vi "Init.vi"(8 "error in (no error)":errorcluster, 11 "optimizer path":path=path "C:/Users/zachc/Documents/Reaction Rover/Plugins/Optimizers/Deep Reaction Optimizer/Source - zmq/start_inference.bat") -> (0 "error out":errorcluster, 3 "optimizer path (out)":path)   [LabVIEW 2020, in "Deep Reaction Optimizer Control Panel.lvlib"]
uses:
  Deep Reaction Optimizer Control Panel.lvlib
  Typedefs/Init.vi States.ctl
panel:
  in  "Connect Btn":bool
  # "1. Optimizer Start Script Path"
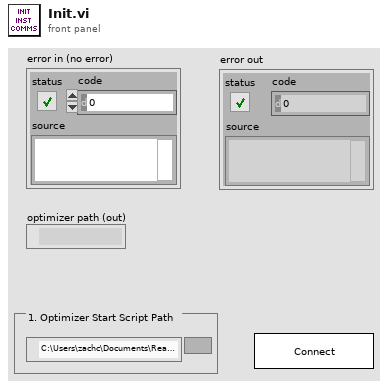
[diagram p1: front panel]
types:
  T1 = typedef "Deep Reaction Optimizer Control Panel.lvlib/Init.vi States.ctl" = enum16{"Waiting for connection", "Connecting", "Successful connection", "Failed to connect", "Closing"}
  T2 = enum32{"Invalid", "Standard", "Closed", "Hidden", "Minimized", "Maximized"}
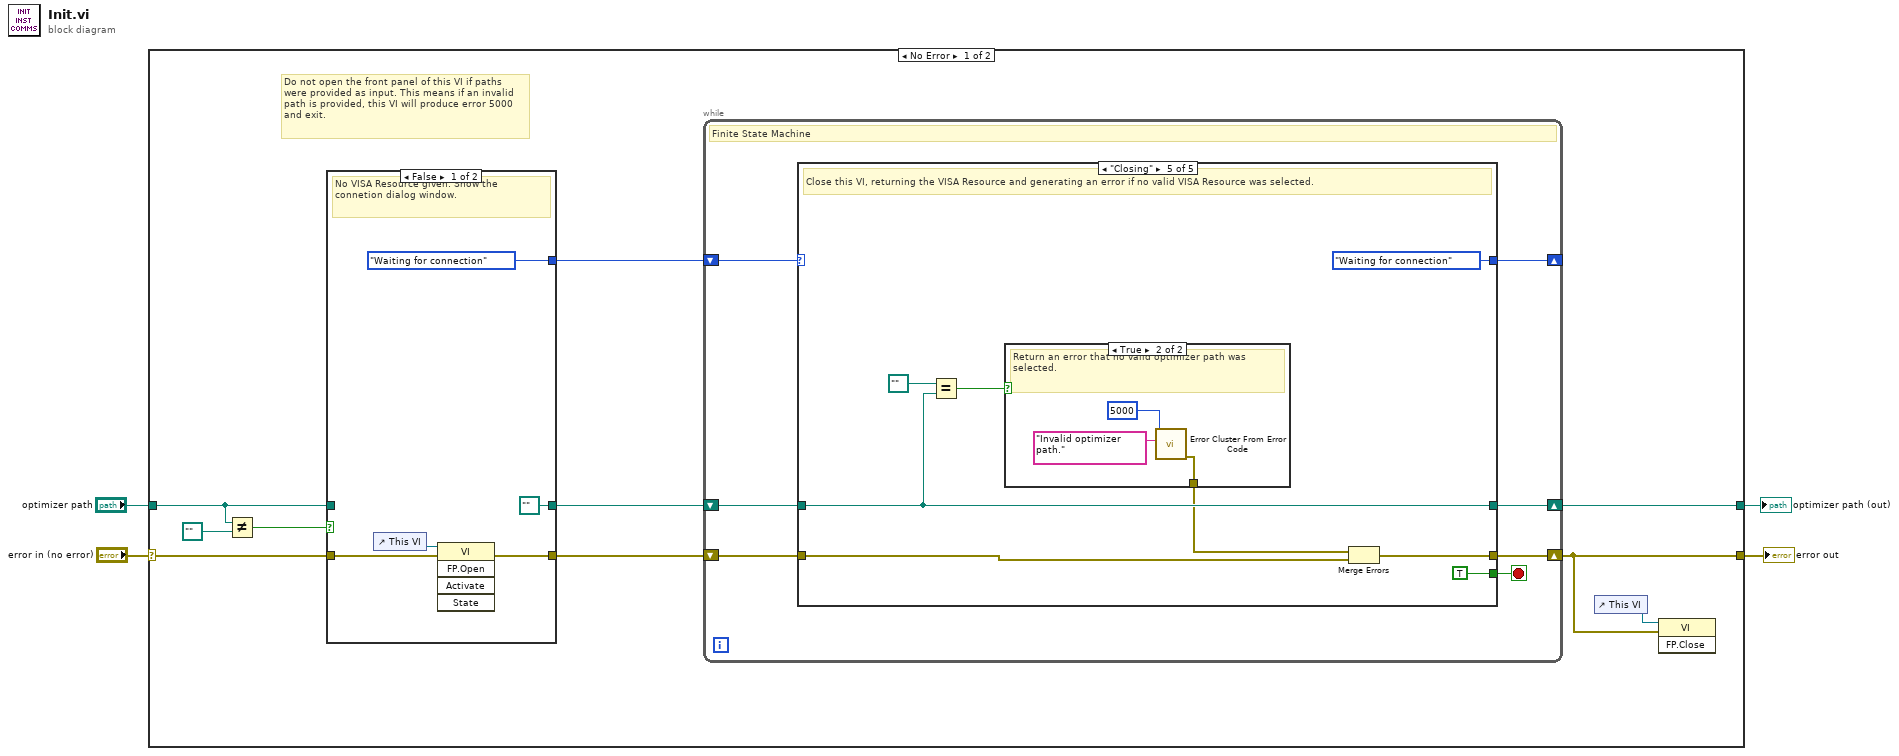
[diagram p0: block diagram]
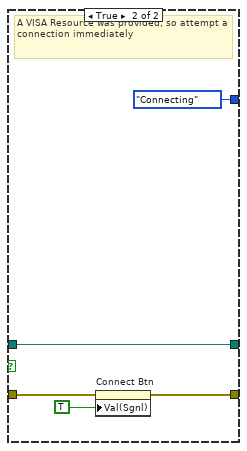
[diagram p2: hidden frame]
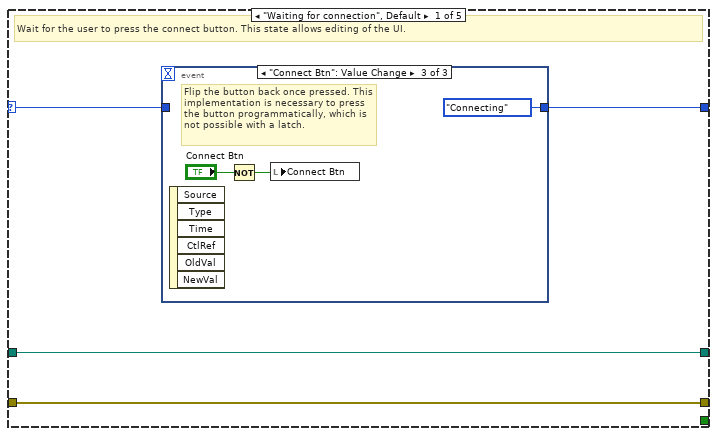
[diagram p3: hidden frame]
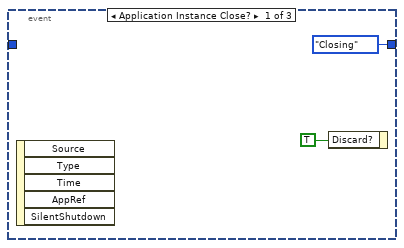
[diagram p4: hidden frame]
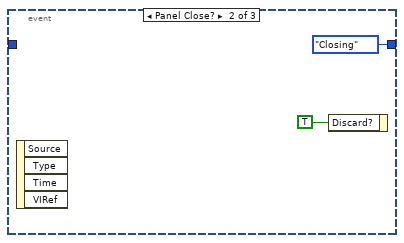
[diagram p5: hidden frame]
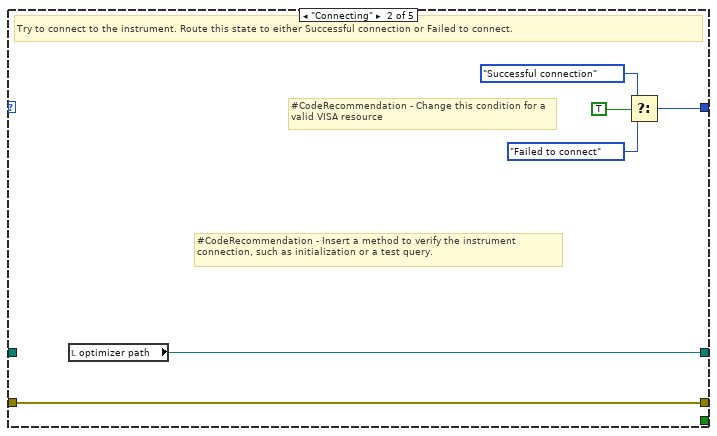
[diagram p6: hidden frame]
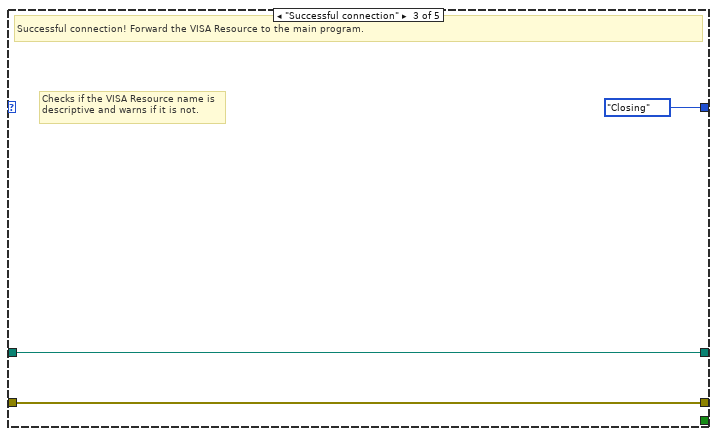
[diagram p7: hidden frame]
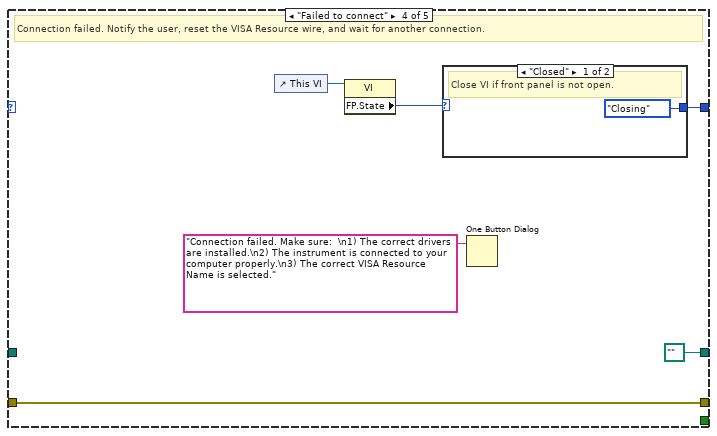
[diagram p8: hidden frame]
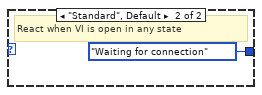
[diagram p9: hidden frame]
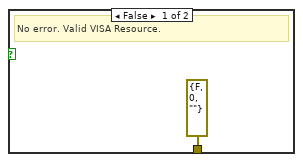
[diagram p10: hidden frame]
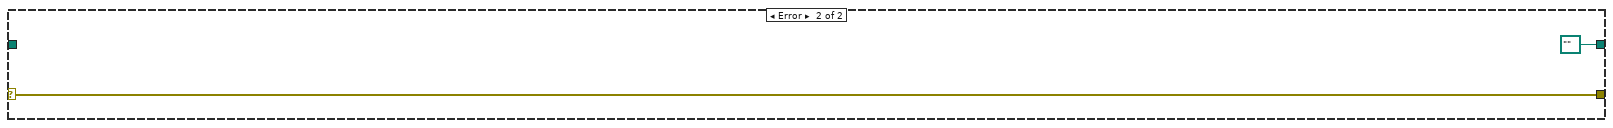
[diagram p11: hidden frame]
diagram:
  n1 = case shown="No Error" "error in (no error)" {
    selector: "error in (no error)" -> [w10 w73]
    tunnel: [w14 path "" ("VISA resource in")] -> w4
    tunnel: [w12 w73] -> w2
    tunnel: "optimizer path" -> [w6 _]
    frame No Error {
      # "Do not open the front panel of this VI if paths were provided as input. This means if an invalid path is provided, this VI will produce error 5000 and exit."
      n2 = Not Equal?(x=w6, y=path "" ("x")) -> (x != y?=w8:bool)
      n3 = case shown="False" w8 {
        tunnel: w10 -> [w18 w23]
        tunnel: [w17 w22] -> w9
        tunnel: [Init.vi_States."Waiting for connection" Init.vi_States."Connecting"] -> w7
        tunnel: w6 -> [_ w20]
        tunnel: [path "" ("optimizer path") w20] -> w5
        frame False {
          # "No VISA Resource given. Show the connetion dialog window."
          n4 = control-ref of="This VI"() -> (w19:refnum<vi>)
          n5 = invoke class="VI" method="FP.Open"(reference=w19, error in=w18) -> (error out=w17:errorcluster)  [unwired: 3 in, 4 out]
        }
        frame True {
          # "A VISA Resource was provided, so attempt a connection immediately"
          n6 = property on="Connect Btn" class="Bool (strict)"(error in=w23, "Val(Sgnl)"=TRUE) -> (error out=w22:errorcluster)  [unwired: 1 in, 1 out]
        }
      }
      n7 = while {
        shift-right: [w30] -> _
        shift-left: w7 -> [w31]
        shift-right: [w28] -> w14
        shift-left: w5 -> [w27]
        shift-right: [w25] -> w12
        shift-left: w9 -> [w26]
        stop <- w29 stop-if-true
        # "Finite State Machine"
        n8 = case shown="\"Closing\"" w31 {
          selector: w31 -> [w35 _ _ _ _]
          tunnel: [w34 w48 Init.vi_States."Closing" w57 Init.vi_States."Waiting for connection"] -> w30
          tunnel: [_ _ _ _ TRUE] -> w29
          tunnel: [w32 w43 w49 path "" ("VISA resource in") w64] -> w28
          tunnel: w27 -> [w32 _ w49 _ w64]
          tunnel: w26 -> [w33 w44 w50 w54 w61]
          tunnel: [w33 w44 w50 w54 w62] -> w25
          frame "Waiting for connection", Default {
            # "Wait for the user to press the connect button. This state allows editing of the UI."
            n9 = event shown="[2] \"Connect Btn\": Value Change" {
              selector: _ -> [_ _ _]
              dyn-events: _ -> [_ _ _]
              timeout: _ -> [_ _ _]
              tunnel: [Init.vi_States."Closing" Init.vi_States."Closing" Init.vi_States."Connecting"] -> w34
              tunnel: w35 -> [_ _ _]
              event Application Instance Close? {
                n10 = event-data() -> ()  [unwired: 1 in, 5 out]
                n11 = event-data("Discard?"=TRUE) -> ()  [unwired: 1 in, 1 out]
              }
              event Panel Close? {
                n12 = event-data() -> ()  [unwired: 1 in, 4 out]
                n13 = event-data("Discard?"=TRUE) -> ()  [unwired: 1 in, 1 out]
              }
              event "Connect Btn": Value Change {
                # "Flip the button back once pressed. This implementation is necessary to press the button programmatically, which is not possible with a latch."
                n14 = event-data() -> ()  [unwired: 1 in, 6 out]
                n15 = Not(x="Connect Btn") -> (.not. x?=w40:bool)
                n16 = local write "Connect Btn"(w40) -> ()
              }
            }
          }
          frame "Connecting" {
            # "#CodeRecommendation - Insert a method to verify the instrument connection, such as initialization or a test query."
            # "#CodeRecommendation - Change this condition for a valid VISA resource"
            # "Try to connect to the instrument. Route this state to either Successful connection or Failed to connect."
            n17 = local read "optimizer path"() -> (w43:path)
            n18 = Select(t=Init.vi_States."Successful connection", s=TRUE, f=Init.vi_States."Failed to connect") -> (s? t:f=w48:T1)
          }
          frame "Successful connection" {
            # "Checks if the VISA Resource name is descriptive and warns if it is not."
            # "Successful connection! Forward the VISA Resource to the main program."
          }
          frame "Failed to connect" {
            # "Connection failed. Notify the user, reset the VISA Resource wire, and wait for another connection."
            n19 = control-ref of="This VI"() -> (w53:refnum<vi>)
            n20 = property class="VI"(reference=w53) -> ("FP.State"=w52:T2)  [unwired: 1 in, 2 out]
            n21 = case shown="\"Closed\"" w52 {
              tunnel: [Init.vi_States."Closing" Init.vi_States."Waiting for connection"] -> w57
              frame "Closed" {
                # "Close VI if front panel is not open."
              }
              frame "Standard", Default {
                # "React when VI is open in any state"
              }
            }
            n22 = One Button Dialog(message="Connection failed. Make sure:  \n1) The correct drivers are installed.\n2) The instrument is connected to your computer properly.\n3) The correct VISA Resource Name is selected.") -> ()  [unwired: 1 in, 1 out]
          }
          frame "Closing" {
            # "Close this VI, returning the VISA Resource and generating an error if no valid VISA Resource was selected."
            n23 = Equal?(x=path "" ("VISA resource in"), y=w64) -> (x = y?=w60:bool)
            n24 = case shown="True" w60 {
              tunnel: [errorcluster {"status"=FALSE, "code"=0, "source"=""} ("error out") w70] -> w63
              frame False {
                # "No error. Valid VISA Resource."
              }
              frame True {
                # "Return an error that no valid optimizer path was selected."
                n25 = call <vilib>:"Error Cluster From Error Code.vi"("error message (\"\")"="Invalid optimizer path." ("error message (\"\")"), "error code (0)"=5000) -> ("error out"=w70:errorcluster)  [unwired: 7 in]
              }
            }
            n26 = Merge Errors(w63, w61) -> (w62:errorcluster)
          }
        }
      }
      n27 = control-ref of="This VI"() -> (w13:refnum<vi>)
      n28 = invoke class="VI" method="FP.Close"(reference=w13, error in=w12) -> ()  [unwired: 1 in, 3 out]
    }
    frame Error {
    }
  }
  "optimizer path (out)" <- w4
  "error out" <- w2
